vi "Find and Validate Function and Device Selection.vi"(7 "reserve?":bool, 8 "error in (no error)":errorcluster, 9 "DevInfos":refnum<class "DevInfo.lvclass">[](array[class]), 10 "Function Name":string, 11 "Controller in":refnum<class "Controller.lvclass">) -> (0 "error out":errorcluster, 1 "Hardware Objects":refnum<class "Hardware.lvclass">[](array[class]), 2 "Function out":refnum<class "Function.lvclass">, 3 "Controller out":refnum<class "Controller.lvclass">)   [LabVIEW 2016, in "Controller Actor.lvlib" / "Controller.lvclass"]
uses:
  <userlib>/Common Components/Controller/Controller.lvclass
  <userlib>/Common Components/Hardware/Abstract Hardware/Hardware.lvclass
  <userlib>/Common Components/Hardware/DevInfo/DevInfo.lvclass
  <userlib>/Common Components/Function Actor/Function.lvclass
  <userlib>/Common Components/Hardware/DevInfo/DevInfo.lvclass/DevInfo.ctl
  <userlib>/Common Components/Controller/Methods/Print List of Hardware (String).vi
  <userlib>/Common Components/Controller/Methods/Print List of Hardware (DevInfo).vi
panel:
  # "INPUTS"
  # "OUTPUTS"
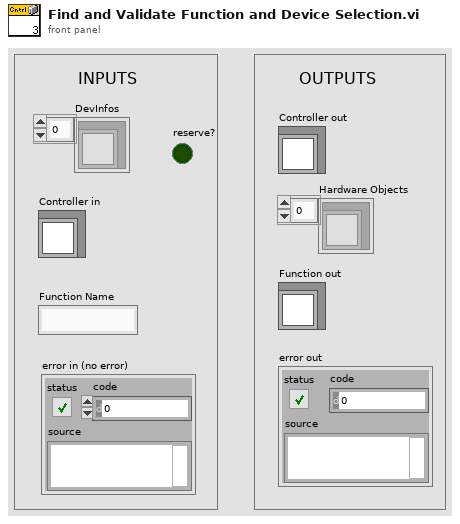
[diagram p1: front panel]
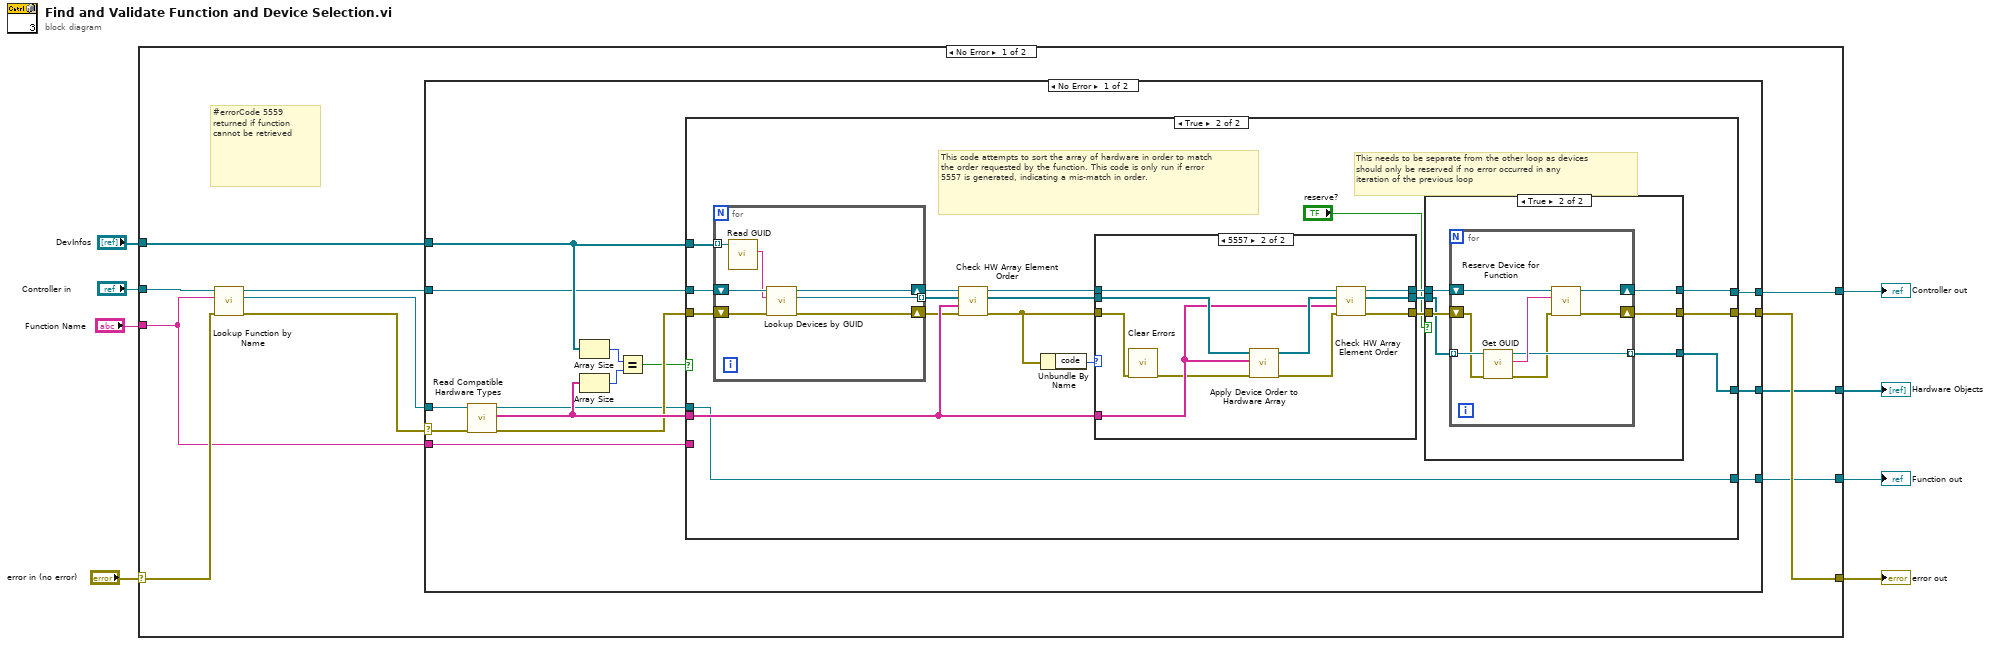
[diagram p0: block diagram]
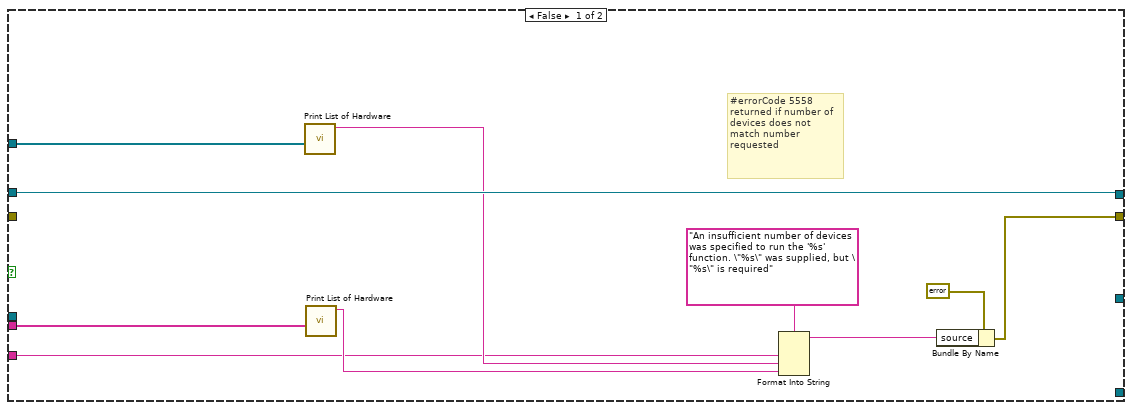
[diagram p2: hidden frame]
diagram:
  n1 = case shown="No Error" "error in (no error)" {
    selector: "error in (no error)" -> [w13 w103]
    tunnel: [w19 w103] -> w8
    tunnel: [w18 w104] -> w7
    tunnel: [w17 _] -> w6
    tunnel: "Controller in" -> [w15 w104]
    tunnel: "DevInfos" -> [w16 _]
    tunnel: "Function Name" -> [w10 _]
    tunnel: [w11 _] -> w2
    frame No Error {
      # "#errorCode 5559 returned if function cannot be retrieved"
      n2 = call <userlib>:"Lookup Function by Name.vi"("error in (no error)"=w13, "Function Name"=w10, "Controller in"=w15) -> ("error out"=w9:errorcluster, "Function.lvclass"=w12:refnum<class "Function.lvclass">, "Controller out"=w14:refnum<class "Controller.lvclass">)  [unwired: 5 in, 1 out]
      n3 = case shown="No Error" w9 {
        selector: w9 -> [w20 w102]
        tunnel: [w34 w102] -> w19
        tunnel: [w33 w101] -> w18
        tunnel: [w32 _] -> w17
        tunnel: w16 -> [w31 _]
        tunnel: w14 -> [w25 w101]
        tunnel: w12 -> [w24 _]
        tunnel: [w22 _] -> w11
        tunnel: w10 -> [w21 _]
        frame No Error {
          n4 = call-dynamic "Read Compatible Hardware Types.vi"("error in (no error)"=w20, "Function in"=w24) -> ("error out"=w29:errorcluster, "Compatible Hardware Types"=w30:string[], "Function out"=w23:refnum<class "Function.lvclass">)  [unwired: 7 in]
          n5 = Array Size(array=w31) -> (size(s)=w27:i32)
          n6 = Array Size(array=w30) -> (size(s)=w26:i32)
          n7 = Equal?(x=w27, y=w26) -> (x = y?=w28:bool)
          n8 = case shown="True" w28 {
            tunnel: [w38 w63] -> w34
            tunnel: [w44 w62] -> w33
            tunnel: [_ w50] -> w32
            tunnel: w29 -> [_ w55]
            tunnel: w25 -> [w44 w57]
            tunnel: w31 -> [w35 w58]
            tunnel: w30 -> [w36 w60]
            tunnel: w23 -> [_ w59]
            tunnel: [_ w59] -> w22
            tunnel: w21 -> [w37 _]
            frame False {
              # "#errorCode 5558 returned if number of devices does not match number requested"
              n9 = call-poly <userlib>:"Print List of Hardware.vi"("Devices"=w35) -> ("String"=w42:string)  [unwired: 10 in]
              n10 = call-poly <userlib>:"Print List of Hardware.vi"("Device Names"=w36) -> ("String"=w41:string)  [unwired: 10 in]
              n11 = Format Into String(format string="An insufficient number of devices was specified to run the '%s' function. \"%s\" was supplied, but \"%s\" is required", w37, w42, w41) -> (resulting string=w39:string)  [unwired: 2 in, 1 out]
              n12 = Bundle By Name(cluster=errorcluster {"status"=TRUE, "code"=5558, "source"=""} ("error out"), "source"=w39) -> (w38:errorcluster)
            }
            frame True {
              # "This code attempts to sort the array of hardware in order to match the order requested by the function. This code is only run if error 5557 is generated, indicating a mis-match in order."
              # "This needs to be separate from the other loop as devices\nshould only be reserved if no error occurred in any\niteration of the previous loop"
              n13 = for {
                tunnel: w58 -> [w99] mode=indexing
                shift-right: [w98] -> w56
                shift-left: w57 -> [w100]
                shift-right: [w96] -> w54
                shift-left: w55 -> [w97]
                tunnel: [w95] -> w53 mode=indexing
                n14 = call <userlib>:"Read GUID.vi"("DevInfo in"=w99) -> ("GUID"=w94:string)  [unwired: 8 in, 2 out]
                n15 = call <userlib>:"Lookup Devices by GUID.vi"("error in (no error)"=w97, "GUID"=w94, "Controller in"=w100) -> ("error out"=w96:errorcluster, "Dev Obj out"=w95:refnum<class "Hardware.lvclass">, "Controller out"=w98:refnum<class "Controller.lvclass">)  [unwired: 6 in]
              }
              n16 = call <userlib>:"Check HW Array Element Order.vi"("error in (no error)"=w54, "Compatible Hardware Types"=w60, "Array of Hardware in"=w53, "Controller in"=w56) -> ("error out"=w48:errorcluster, "Array of Hardware out"=w49:refnum<class "Hardware.lvclass">[], "Controller out"=w46:refnum<class "Controller.lvclass">)  [unwired: 5 in]
              n17 = Unbundle By Name(w48) -> ("code"=w47:i32)
              n18 = case shown="5557" w47 {
                tunnel: w60 -> [_ w89]
                tunnel: w49 -> [w82 w93]
                tunnel: [w83 w86] -> w52
                tunnel: w48 -> [w83 w84]
                tunnel: w46 -> [w81 w92]
                tunnel: [w81 w91] -> w61
                tunnel: [w82 w88] -> w51
                frame Default {
                }
                frame 5557 {
                  n19 = call <vilib>:"Clear Errors.vi"("error in (no error)"=w84) -> ("error out"=w85:errorcluster)  [unwired: 5 in, 1 out]
                  n20 = call <userlib>:"Apply Device Order to Hardware Array.vi"("error in (no error)"=w85, "Compatible Hardware Types"=w89, "Array of Hardware in"=w93) -> ("error out"=w87:errorcluster, "Array"=w90:refnum<class "Hardware.lvclass">[])  [unwired: 7 in]
                  n21 = call <userlib>:"Check HW Array Element Order.vi"("error in (no error)"=w87, "Compatible Hardware Types"=w89, "Array of Hardware in"=w90, "Controller in"=w92) -> ("error out"=w86:errorcluster, "Array of Hardware out"=w88:refnum<class "Hardware.lvclass">[], "Controller out"=w91:refnum<class "Controller.lvclass">)  [unwired: 5 in]
                }
              }
              n22 = case shown="True" "reserve?" {
                tunnel: [w65 w72] -> w63
                tunnel: [w66 w71] -> w62
                tunnel: w61 -> [w66 w70]
                tunnel: w52 -> [w65 w69]
                tunnel: w51 -> [w64 w68]
                tunnel: [w64 w67] -> w50
                frame False {
                }
                frame True {
                  n23 = for {
                    shift-right: [w79] -> w71
                    shift-left: w70 -> [w80]
                    shift-right: [w78] -> w72
                    shift-left: w69 -> [w74]
                    tunnel: w68 -> [w77] mode=indexing
                    tunnel: [w75] -> w67 mode=indexing
                    n24 = call <userlib>:"Get GUID.vi"("error in (no error)"=w74, "Hardware in"=w77) -> ("error out"=w73:errorcluster, "GUID"=w76:string, "Hardware out"=w75:refnum<class "Hardware.lvclass">)  [unwired: 7 in]
                    n25 = call <userlib>:"Reserve Device for Function.vi"("error in (no error)"=w73, "Device (GUID) to Reserve"=w76, "Controller in"=w80) -> ("error out"=w78:errorcluster, "Controller out"=w79:refnum<class "Controller.lvclass">)  [unwired: 7 in]
                  }
                }
              }
            }
          }
        }
        frame Error {
        }
      }
    }
    frame Error {
    }
  }
  "error out" <- w8
  "Controller out" <- w7
  "Hardware Objects" <- w6
  "Function out" <- w2
